vi "run_pipeline.vi"(0 "data_simple_pipeline in":refnum<class "data_simple_pipeline.lvclass">, 11 "error in (no error)":errorcluster) -> (4 "data_simple_pipeline out":refnum<class "data_simple_pipeline.lvclass">, 15 "error out":errorcluster)   [LabVIEW 2020, in "data_simple_pipeline.lvclass"]
uses:
  data_simple_pipeline.lvclass
  data_simple_pipeline.lvclass/data_simple_pipeline.ctl
  data/data_document/data_document.lvclass
  D:/Personal/LabVIEW LLMs/src/data/abstract_data_base/abstract_data_base.lvclass
  data/data_node/data_node.lvclass
  data_source/abstract_datasource_base/abstract_datasource_base.lvclass
  data_processor/abstract_dataprocessing_base/abstract_dataprocessing_base.lvclass
  data_destination/abstract_datadestination_base/abstract_datadestination_base.lvclass
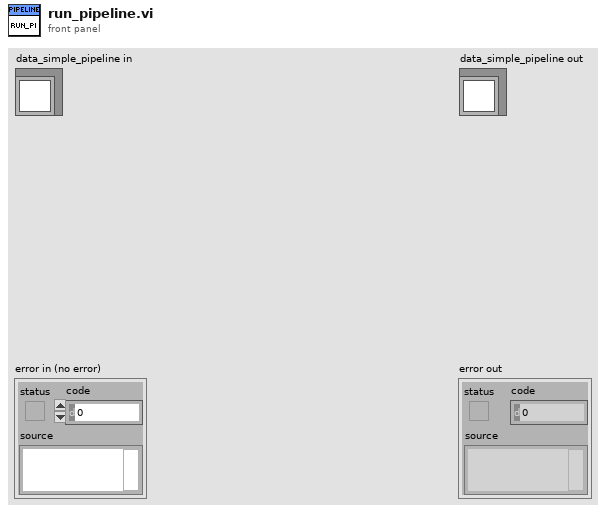
[diagram p1: front panel]
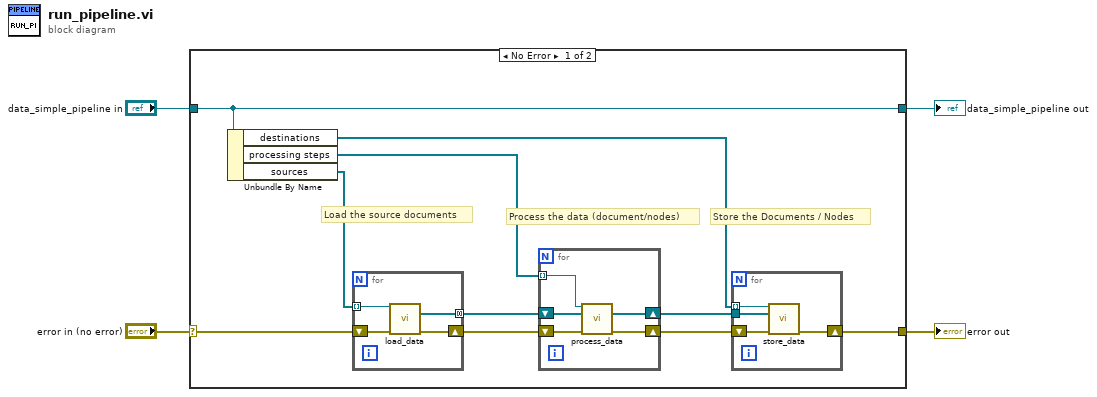
[diagram p0: block diagram]
diagram:
  n1 = case shown="No Error" "error in (no error)" {
    selector: "error in (no error)" -> [w12 w29]
    tunnel: [w6 w29] -> w3
    tunnel: [w14 w28] -> w1
    tunnel: "data_simple_pipeline in" -> [w14 w28]
    frame No Error {
      # "Store the Documents / Nodes"
      # "Process the data (document/nodes)"
      # "Load the source documents"
      n2 = Unbundle By Name(w14) -> ("destinations"=w7:refnum<class "abstract_datadestination_base.lvclass">[], "processing steps"=w10:refnum<class "abstract_dataprocessing_base.lvclass">[], "sources"=w13:refnum<class "abstract_datasource_base.lvclass">[])
      n3 = for {
        tunnel: w13 -> [w27] mode=indexing
        tunnel: [w25] -> w9 mode=concatenating
        shift-right: [w24] -> w11
        shift-left: w12 -> [w26]
        n4 = call-dynamic "load_data.vi"("abstract_datasource_base in"=w27, "error in (no error)"=w26) -> ("document"=w25:refnum<class "data_document.lvclass">[], "error out"=w24:errorcluster)  [unwired: 11 in, 1 out]
      }
      n5 = for {
        tunnel: w10 -> [w21] mode=indexing
        shift-right: [w22] -> w8
        shift-left: w11 -> [w23]
        shift-right: [w19] -> w5
        shift-left: w9 -> [w20]
        n6 = call-dynamic "process_data.vi"("abstract_dataprocessing_base in"=w21, "datas"=w20, "error in (no error)"=w23) -> ("nodes"=w19:refnum<class "data_node.lvclass">[], "error out"=w22:errorcluster)  [unwired: 10 in, 1 out]
      }
      n7 = for {
        tunnel: w7 -> [w18] mode=indexing
        shift-right: [w16] -> w6
        shift-left: w8 -> [w17]
        tunnel: w5 -> [w15]
        n8 = call-dynamic "store_data.vi"("abstract_datadestination_base in"=w18, "datas"=w15, "error in (no error)"=w17) -> ("error out"=w16:errorcluster)  [unwired: 11 in, 1 out]
      }
    }
    frame Error {
    }
  }
  "error out" <- w3
  "data_simple_pipeline out" <- w1
